vi "PathPlanner_Cmd_FollowHolonomicPathPack.vi"(0 "Rotation Tolerance DEG":dbl=0.0872665, 1 "Trigger Events":bool=TRUE, 4 "Y Tolerance M":dbl=0.0762, 5 "HOLONOMIC_CTRL_PACK_TUNING":T2={"X PID Tuning"={"Kp"=0.0, "Ki"=0.0, "Kd"=0.0, "MaximumIntegral"=9.9e+30, "MinimumIntegral"=-9.9e+30}, "Y PID Tuning"={"Kp"=0.0, "Ki"=0.0, "Kd"=0.0, "MaximumIntegral"=9.9e+30, "MinimumIntegral"=-9.9e+30}, "thetaProfiledPID_CTRL"={"Controller"={"Kp"=0.0, "Ki"=0.0, "Kd"=0.0, "Period"=0.0, "Max_Integral"=1.0, "Min_Integral"=-1.0, "Max_Input"=0.0, "Min_Input"=0.0, "Continuous"=FALSE, "PositionError"=0.0, "VelocityError"=0.0, "PrevError"=0.0, "TotalError"=0.0, "PositionTolerance"=0.05, "VelocityTolerance"=9.99e+35, "SetPoint"=0.0, "Kf"=0.0, "Prev_Deriv"=0.0, "Prev_Deriv 2"=0.0, "DerivativeFilter"=FALSE, "Min_Output"=-9.99e+35, "Max_Output"=9.9e+35, "Prev_F_P"=0.0, "Prev_F_P_2"=0.0, "AntiWindupActive"=FALSE, "Measurement"=0.0}, "Goal"={"Position"=0.0, "Velocity"=0.0}, "Setpoint"={"Position"=0.0, "Velocity"=0.0}, "Constraint"={"MaxVelocity"=0.0, "MaxAcceleration"=0.0}}} {"thetaProfiledPID_CTRL"."Constraint"."MaxAcceleration" format="%16_6e"; "thetaProfiledPID_CTRL"."Constraint"."MaxVelocity" format="%16_6e"; "thetaProfiledPID_CTRL"."Setpoint"."Velocity" format="%16_6e"; "thetaProfiledPID_CTRL"."Setpoint"."Position" format="%16_6e"; "thetaProfiledPID_CTRL"."Goal"."Velocity" format="%16_6e"; "thetaProfiledPID_CTRL"."Goal"."Position" format="%16_6e"; "thetaProfiledPID_CTRL"."Controller"."Measurement" format="%16_6e"; "thetaProfiledPID_CTRL"."Controller"."Prev_F_P_2" format="%16_6e"; "thetaProfiledPID_CTRL"."Controller"."Prev_F_P" format="%16_6e"; "thetaProfiledPID_CTRL"."Controller"."Max_Output" format="%16_6e"; "thetaProfiledPID_CTRL"."Controller"."Min_Output" format="%16_6e"; "thetaProfiledPID_CTRL"."Controller"."Prev_Deriv 2" format="%16_6e"; "thetaProfiledPID_CTRL"."Controller"."Prev_Deriv" format="%16_6e"; "thetaProfiledPID_CTRL"."Controller"."Kf" format="%16_6e"; "thetaProfiledPID_CTRL"."Controller"."SetPoint" format="%16_6e"; "thetaProfiledPID_CTRL"."Controller"."VelocityTolerance" format="%16_6e"; "thetaProfiledPID_CTRL"."Controller"."PositionTolerance" format="%16_6e"; "thetaProfiledPID_CTRL"."Controller"."TotalError" format="%16_6e"; "thetaProfiledPID_CTRL"."Controller"."PrevError" format="%16_6e"; "thetaProfiledPID_CTRL"."Controller"."VelocityError" format="%16_6e"; "thetaProfiledPID_CTRL"."Controller"."PositionError" format="%16_6e"; "thetaProfiledPID_CTRL"."Controller"."Min_Input" format="%16_6e"; "thetaProfiledPID_CTRL"."Controller"."Max_Input" format="%16_6e"; "thetaProfiledPID_CTRL"."Controller"."Min_Integral" format="%16_6e"; "thetaProfiledPID_CTRL"."Controller"."Max_Integral" format="%16_6e"; "thetaProfiledPID_CTRL"."Controller"."Period" format="%16_6e"; "thetaProfiledPID_CTRL"."Controller"."Kd" format="%16_6e"; "thetaProfiledPID_CTRL"."Controller"."Ki" format="%16_6e"; "thetaProfiledPID_CTRL"."Controller"."Kp" format="%16_6e"}, 6 "X Tolerance M":dbl=0.0762, 7 "ReplanningConfig":T1={"enableInitialReplanning"=TRUE, "enableDynamicReplanning"=FALSE, "dynamicReplanningTotalErrorThreshold"=1.0, "dynamicReplanningErrorSpikeThreshold"=0.25}, 8 "ControlPastEnd_Sec":dbl=3.0, 9 "Period_Sec":dbl=0.02, 10 "Drive Base Radius M":dbl, 11 "Max Wheel Speed M/S":dbl) -> (3 "PathPlanner_Ctrl_HolDrvConfig":T8={"HOLONOMIC_CTRL_PACK_TUNING"={"X PID Tuning"={"Kp"=0.0, "Ki"=0.0, "Kd"=0.0, "MaximumIntegral"=9.9e+30, "MinimumIntegral"=-9.9e+30}, "Y PID Tuning"={"Kp"=0.0, "Ki"=0.0, "Kd"=0.0, "MaximumIntegral"=9.9e+30, "MinimumIntegral"=-9.9e+30}, "thetaProfiledPID_CTRL"={"Controller"={"Kp"=0.0, "Ki"=0.0, "Kd"=0.0, "Period"=0.0, "Max_Integral"=1.0, "Min_Integral"=-1.0, "Max_Input"=0.0, "Min_Input"=0.0, "Continuous"=FALSE, "PositionError"=0.0, "VelocityError"=0.0, "PrevError"=0.0, "TotalError"=0.0, "PositionTolerance"=0.05, "VelocityTolerance"=9.99e+35, "SetPoint"=0.0, "Kf"=0.0, "Prev_Deriv"=0.0, "Prev_Deriv 2"=0.0, "DerivativeFilter"=FALSE, "Min_Output"=-9.99e+35, "Max_Output"=9.9e+35, "Prev_F_P"=0.0, "Prev_F_P_2"=0.0, "AntiWindupActive"=FALSE, "Measurement"=0.0}, "Goal"={"Position"=0.0, "Velocity"=0.0}, "Setpoint"={"Position"=0.0, "Velocity"=0.0}, "Constraint"={"MaxVelocity"=0.0, "MaxAcceleration"=0.0}}}, "Max Wheel Speed M/S"=0.0, "Tolerance SI"={"TRANSLATION"={"X"=0.04, "Y"=0.04}, "ROTATION"={"VALUE"=0.034906585039887, "COS"=0.999390827019096, "SIN"=0.034899496702501}}, "Drive Base Radius M"=0.0, "ControlPastEnd_Sec"=3.0, "ReplanningConfig"={"enableInitialReplanning"=FALSE, "enableDynamicReplanning"=FALSE, "dynamicReplanningTotalErrorThreshold"=0.0, "dynamicReplanningErrorSpikeThreshold"=0.0}, "Period_Sec"=0.02, "Trigger Events"=TRUE} {"Tolerance SI"."ROTATION"."SIN" format="%13.4f"; "Tolerance SI"."ROTATION"."COS" format="%13.4f"; "Tolerance SI"."ROTATION"."VALUE" format="%13.4f"; "Tolerance SI"."TRANSLATION"."Y" format="%14.3f"; "Tolerance SI"."TRANSLATION"."X" format="%14.3f"; "HOLONOMIC_CTRL_PACK_TUNING"."thetaProfiledPID_CTRL"."Constraint"."MaxAcceleration" format="%16_6e"; "HOLONOMIC_CTRL_PACK_TUNING"."thetaProfiledPID_CTRL"."Constraint"."MaxVelocity" format="%16_6e"; "HOLONOMIC_CTRL_PACK_TUNING"."thetaProfiledPID_CTRL"."Setpoint"."Velocity" format="%16_6e"; "HOLONOMIC_CTRL_PACK_TUNING"."thetaProfiledPID_CTRL"."Setpoint"."Position" format="%16_6e"; "HOLONOMIC_CTRL_PACK_TUNING"."thetaProfiledPID_CTRL"."Goal"."Velocity" format="%16_6e"; "HOLONOMIC_CTRL_PACK_TUNING"."thetaProfiledPID_CTRL"."Goal"."Position" format="%16_6e"; "HOLONOMIC_CTRL_PACK_TUNING"."thetaProfiledPID_CTRL"."Controller"."Measurement" format="%16_6e"; "HOLONOMIC_CTRL_PACK_TUNING"."thetaProfiledPID_CTRL"."Controller"."Prev_F_P_2" format="%16_6e"; "HOLONOMIC_CTRL_PACK_TUNING"."thetaProfiledPID_CTRL"."Controller"."Prev_F_P" format="%16_6e"; "HOLONOMIC_CTRL_PACK_TUNING"."thetaProfiledPID_CTRL"."Controller"."Max_Output" format="%16_6e"; "HOLONOMIC_CTRL_PACK_TUNING"."thetaProfiledPID_CTRL"."Controller"."Min_Output" format="%16_6e"; "HOLONOMIC_CTRL_PACK_TUNING"."thetaProfiledPID_CTRL"."Controller"."Prev_Deriv 2" format="%16_6e"; "HOLONOMIC_CTRL_PACK_TUNING"."thetaProfiledPID_CTRL"."Controller"."Prev_Deriv" format="%16_6e"; "HOLONOMIC_CTRL_PACK_TUNING"."thetaProfiledPID_CTRL"."Controller"."Kf" format="%16_6e"; "HOLONOMIC_CTRL_PACK_TUNING"."thetaProfiledPID_CTRL"."Controller"."SetPoint" format="%16_6e"; "HOLONOMIC_CTRL_PACK_TUNING"."thetaProfiledPID_CTRL"."Controller"."VelocityTolerance" format="%16_6e"; "HOLONOMIC_CTRL_PACK_TUNING"."thetaProfiledPID_CTRL"."Controller"."PositionTolerance" format="%16_6e"; "HOLONOMIC_CTRL_PACK_TUNING"."thetaProfiledPID_CTRL"."Controller"."TotalError" format="%16_6e"; "HOLONOMIC_CTRL_PACK_TUNING"."thetaProfiledPID_CTRL"."Controller"."PrevError" format="%16_6e"; "HOLONOMIC_CTRL_PACK_TUNING"."thetaProfiledPID_CTRL"."Controller"."VelocityError" format="%16_6e"; "HOLONOMIC_CTRL_PACK_TUNING"."thetaProfiledPID_CTRL"."Controller"."PositionError" format="%16_6e"; "HOLONOMIC_CTRL_PACK_TUNING"."thetaProfiledPID_CTRL"."Controller"."Min_Input" format="%16_6e"; "HOLONOMIC_CTRL_PACK_TUNING"."thetaProfiledPID_CTRL"."Controller"."Max_Input" format="%16_6e"; "HOLONOMIC_CTRL_PACK_TUNING"."thetaProfiledPID_CTRL"."Controller"."Min_Integral" format="%16_6e"; "HOLONOMIC_CTRL_PACK_TUNING"."thetaProfiledPID_CTRL"."Controller"."Max_Integral" format="%16_6e"; "HOLONOMIC_CTRL_PACK_TUNING"."thetaProfiledPID_CTRL"."Controller"."Period" format="%16_6e"; "HOLONOMIC_CTRL_PACK_TUNING"."thetaProfiledPID_CTRL"."Controller"."Kd" format="%16_6e"; "HOLONOMIC_CTRL_PACK_TUNING"."thetaProfiledPID_CTRL"."Controller"."Ki" format="%16_6e"; "HOLONOMIC_CTRL_PACK_TUNING"."thetaProfiledPID_CTRL"."Controller"."Kp" format="%16_6e"})   [LabVIEW 2019, in "PathPlanner24.lvlib"]
doc: "DOCUMENTATION IS NOT COMPLETE.\n \nPack controller tuning configuration for Path Planner Holonomic Drive Controller.\n\nInputs:\n - X PID Tuning - cluster - Input from PACK PROF PID VI\n - Y PID Tuning - cluster - Input from PACK PROF PID VI\n - thetaController - cluster - A profiled PID controller to respond to error in angle.\n - Max Wheel Speed M/.S - double - Maximum wheel speed (M/S)\n - DriveBaseRadius - double - The radius of the drive base in meters. For swerve drive, this is the\n distance from the center of the robot to the furthest module. For \n mecanum, this is the drive base width / 2\n - X Tolerance - double - X tolerance for calculating At Reference (Meters) (Optional. Default: 0.0762 )\n - Y Tolerance - double - Y tolerance for calculating At Reference (Meters) (Optional. Default: 0.0762 )\n - Rotation Tolerance - double - Rotation tolerance for calculating At Reference (Degrees) (Optional. Default: 0.0)873)\n\nOutputs:\n -- PathPlannerHolCtrlConfig -- cluster - packed controller configuration."
uses:
  PathPlanner24.lvlib
  TypeDef/PathPlannerCmdFollowHolConfig.ctl
  <vilib>/Rock Robotics/WPI/ThirdParty/JAS_Junk/TrajLib/TypeDef/HOLONOMIC_PACK_TUNING.ctl
  <vilib>/Rock Robotics/WPI/ThirdParty/JAS_Junk/TrajLib/TypeDef/PID_TUNING.ctl
  <vilib>/Rock Robotics/WPI/ThirdParty/JAS_Junk/TrajLib/TypeDef/PROFILED_PID_CONTROLLER.ctl
  <vilib>/Rock Robotics/WPI/ThirdParty/JAS_Junk/TrajLib/TypeDef/PID_CONTROLLER.ctl
  <vilib>/Rock Robotics/WPI/ThirdParty/JAS_Junk/TrajLib/TypeDef/TRAPEZOID_PROFILE_STATE.ctl
  <vilib>/Rock Robotics/WPI/ThirdParty/JAS_Junk/TrajLib/TypeDef/TRAPEZOID_PROFILE_CONSTRAINT.ctl
  <vilib>/Rock Robotics/WPI/ThirdParty/JAS_Junk/TrajLib/TypeDef/POSE2D.ctl
  <vilib>/Rock Robotics/WPI/ThirdParty/JAS_Junk/TrajLib/TypeDef/TRANSLATION2D.ctl
  <vilib>/Rock Robotics/WPI/ThirdParty/JAS_Junk/TrajLib/TypeDef/ROTATION2D.ctl
  TypeDef/PathPlannerReplanningConfig.ctl
  <vilib>/Rock Robotics/WPI/ThirdParty/JAS_Junk/TrajLib/Rotation2d_CreateAngle.vi
  <vilib>/Rock Robotics/WPI/ThirdParty/JAS_Junk/TrajLib/Translation2d_Create.vi
  <vilib>/Rock Robotics/WPI/ThirdParty/JAS_Junk/TrajLib/Trajectory_Library.lvlib
panel:
  # "3 inches"
  # "5 deg"
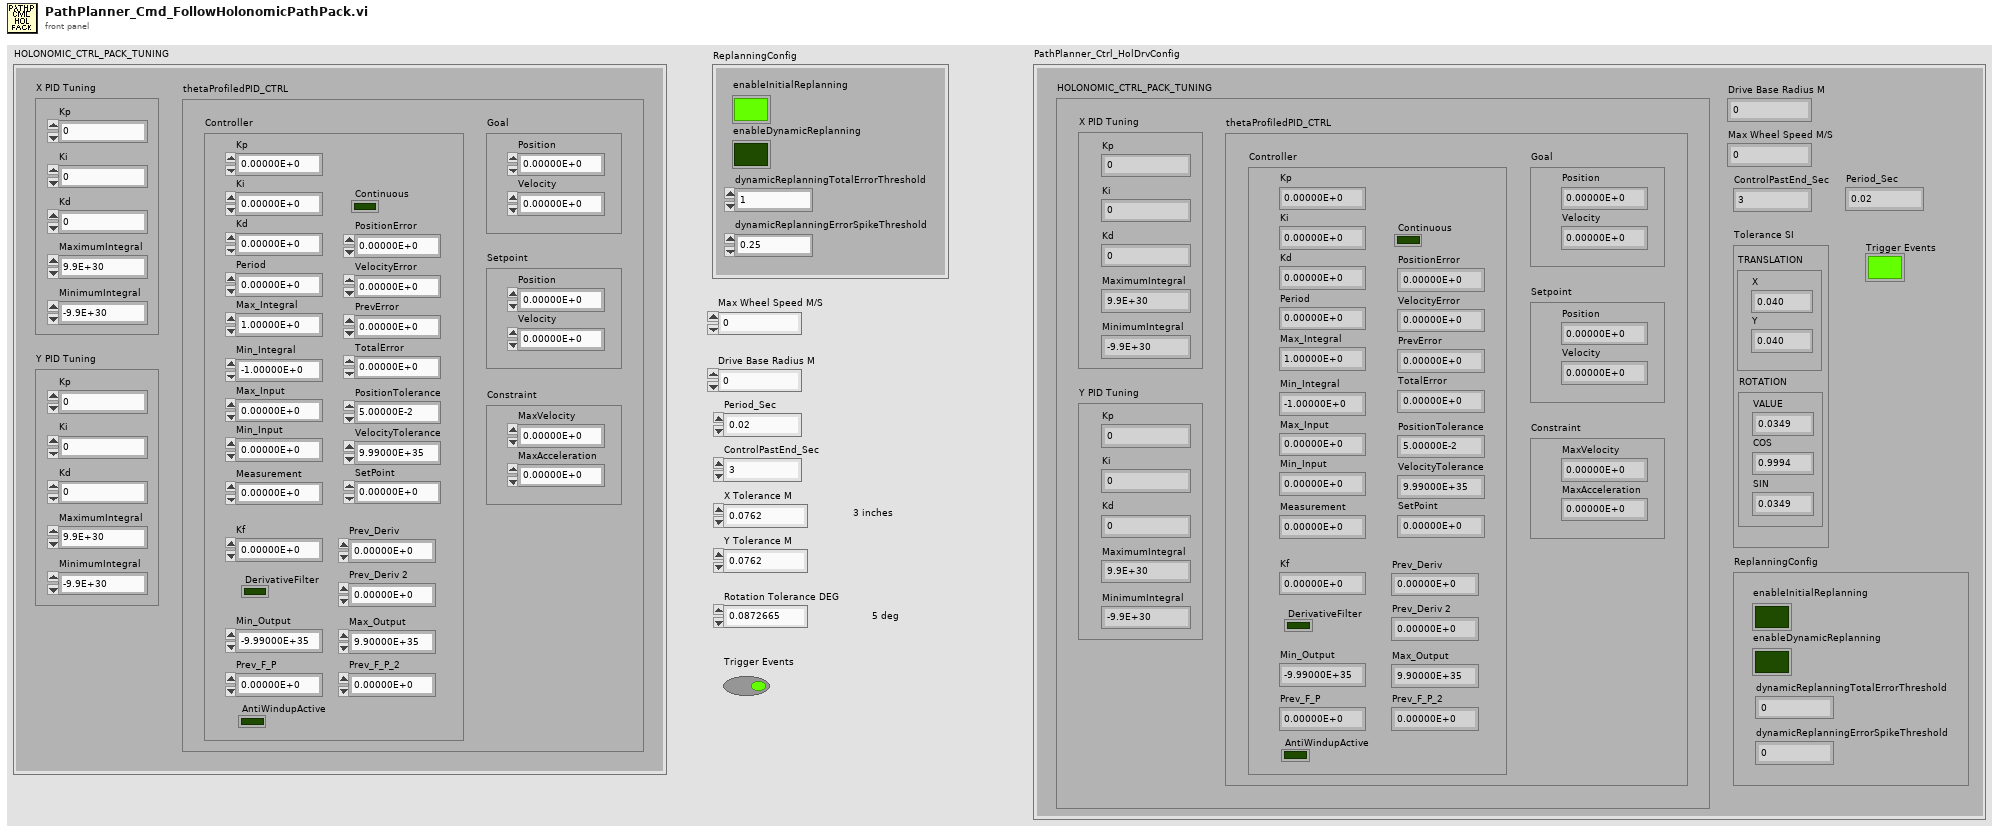
[diagram p1: front panel]
types:
  T1 = typedef "PathPlanner24.lvlib/PathPlannerReplanningConfig.ctl" = cluster{"enableInitialReplanning":bool, "enableDynamicReplanning":bool, "dynamicReplanningTotalErrorThreshold":dbl, "dynamicReplanningErrorSpikeThreshold":dbl}
  T2 = typedef "Trajectory_Library.lvlib/HOLONOMIC_PACK_TUNING.ctl" = cluster{"X PID Tuning":T3, "Y PID Tuning":T3, "thetaProfiledPID_CTRL":T4}
  T3 = typedef "Trajectory_Library.lvlib/PID_TUNING.ctl" = cluster{"Kp":dbl, "Ki":dbl, "Kd":dbl, "MaximumIntegral":dbl, "MinimumIntegral":dbl}
  T4 = typedef "Trajectory_Library.lvlib/PROFILED_PID_CONTROLLER.ctl" = cluster{"Controller":T5, "Goal":T6, "Setpoint":T6, "Constraint":T7}
  T5 = typedef "Trajectory_Library.lvlib/PID_CONTROLLER.ctl" = cluster{"Kp":dbl, "Ki":dbl, "Kd":dbl, "Period":dbl, "Max_Integral":dbl, "Min_Integral":dbl, "Max_Input":dbl, "Min_Input":dbl, "Continuous":bool, "PositionError":dbl, "VelocityError":dbl, "PrevError":dbl, "TotalError":dbl, "PositionTolerance":dbl, "VelocityTolerance":dbl, "SetPoint":dbl, "Kf":dbl, "Prev_Deriv":dbl, "Prev_Deriv 2":dbl, "DerivativeFilter":bool, "Min_Output":dbl, "Max_Output":dbl, "Prev_F_P":dbl, "Prev_F_P_2":dbl, "AntiWindupActive":bool, "Measurement":dbl}
  T6 = typedef "Trajectory_Library.lvlib/TRAPEZOID_PROFILE_STATE.ctl" = cluster{"Position":dbl, "Velocity":dbl}
  T7 = typedef "Trajectory_Library.lvlib/TRAPEZOID_PROFILE_CONSTRAINT.ctl" = cluster{"MaxVelocity":dbl, "MaxAcceleration":dbl}
  T8 = typedef "PathPlanner24.lvlib/PathPlannerCmdFollowHolConfig.ctl" = cluster{"HOLONOMIC_CTRL_PACK_TUNING":T2, "Max Wheel Speed M/S":dbl, "Tolerance SI":T9, "Drive Base Radius M":dbl, "ControlPastEnd_Sec":dbl, "ReplanningConfig":T1, "Period_Sec":dbl, "Trigger Events":bool}
  T9 = typedef "Trajectory_Library.lvlib/POSE2D.ctl" = cluster{"TRANSLATION":T10, "ROTATION":T11}
  T10 = typedef "Trajectory_Library.lvlib/TRANSLATION2D.ctl" = cluster{"X":dbl, "Y":dbl}
  T11 = typedef "Trajectory_Library.lvlib/ROTATION2D.ctl" = cluster{"VALUE":dbl, "COS":dbl, "SIN":dbl}
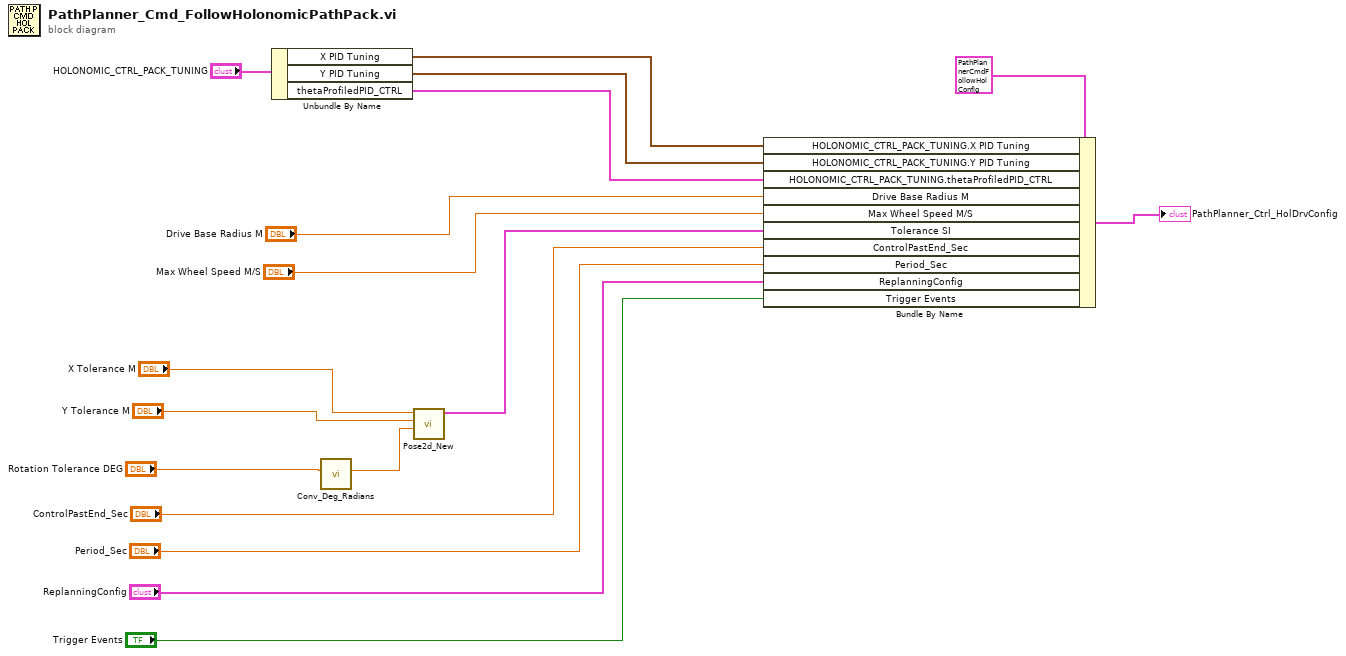
[diagram p0: block diagram]
diagram:
  n1 = Unbundle By Name("HOLONOMIC_CTRL_PACK_TUNING") -> ("X PID Tuning"=w8:T3, "Y PID Tuning"=w7:T3, "thetaProfiledPID_CTRL"=w6:T4)
  n2 = call <vilib>:"Conv_Deg_Radians.vi"("Degress"="Rotation Tolerance DEG") -> ("Radians"=w15:dbl)  [unwired: 10 in]
  n3 = call <vilib>:"Pose2d_New.vi"("Heading"=w15, "Y"="Y Tolerance M", "X"="X Tolerance M") -> ("out POSe"=w11:T9)  [unwired: 8 in]
  n4 = Bundle By Name(cluster=T8 {"HOLONOMIC_CTRL_PACK_TUNING"={"X PID Tuning"={"Kp"=0.0, "Ki"=0.0, "Kd"=0.0, "MaximumIntegral"=9.9e+30, "MinimumIntegral"=-9.9e+30}, "Y PID Tuning"={"Kp"=0.0, "Ki"=0.0, "Kd"=0.0, "MaximumIntegral"=9.9e+30, "MinimumIntegral"=-9.9e+30}, "thetaProfiledPID_CTRL"={"Controller"={"Kp"=0.0, "Ki"=0.0, "Kd"=0.0, "Period"=0.0, "Max_Integral"=1.0, "Min_Integral"=-1.0, "Max_Input"=0.0, "Min_Input"=0.0, "Continuous"=FALSE, "PositionError"=0.0, "VelocityError"=0.0, "PrevError"=0.0, "TotalError"=0.0, "PositionTolerance"=0.05, "VelocityTolerance"=9.99e+35, "SetPoint"=0.0, "Kf"=0.0, "Prev_Deriv"=0.0, "Prev_Deriv 2"=0.0, "DerivativeFilter"=FALSE, "Min_Output"=-9.99e+35, "Max_Output"=9.9e+35, "Prev_F_P"=0.0, "Prev_F_P_2"=0.0, "AntiWindupActive"=FALSE, "Measurement"=0.0}, "Goal"={"Position"=0.0, "Velocity"=0.0}, "Setpoint"={"Position"=0.0, "Velocity"=0.0}, "Constraint"={"MaxVelocity"=0.0, "MaxAcceleration"=0.0}}}, "Max Wheel Speed M/S"=0.0, "Tolerance SI"={"TRANSLATION"={"X"=0.04, "Y"=0.04}, "ROTATION"={"VALUE"=0.034906585039887, "COS"=0.999390827019096, "SIN"=0.034899496702501}}, "Drive Base Radius M"=0.0, "ControlPastEnd_Sec"=3.0, "ReplanningConfig"={"enableInitialReplanning"=TRUE, "enableDynamicReplanning"=FALSE, "dynamicReplanningTotalErrorThreshold"=1.0, "dynamicReplanningErrorSpikeThreshold"=0.25}, "Period_Sec"=0.02, "Trigger Events"=TRUE} ("PathPlanner_Cmd_FollowHolConfig"), "HOLONOMIC_CTRL_PACK_TUNING.X PID Tuning"=w8, "HOLONOMIC_CTRL_PACK_TUNING.Y PID Tuning"=w7, "HOLONOMIC_CTRL_PACK_TUNING.thetaProfiledPID_CTRL"=w6, "Drive Base Radius M"="Drive Base Radius M", "Max Wheel Speed M/S"="Max Wheel Speed M/S", "Tolerance SI"=w11, "ControlPastEnd_Sec"="ControlPastEnd_Sec", "Period_Sec"="Period_Sec", "ReplanningConfig"="ReplanningConfig", "Trigger Events"="Trigger Events") -> (→"PathPlanner_Ctrl_HolDrvConfig":T8)
